vi "Master Setup Get Label and Pattern.vi"(2 "Use Master Setup":bool, 3 "Master Setup Patten Enum":i32(ring) items=["Channel Setup (0)", "PID Setup (1)", "Filter Setup (2)", "CAN Message Setup (3)", "CAN 1 Setup (4)", "CAN 2 Setup (5)", "Digital Inputs Setup (6)", "Digital Outputs Setup (7)", "Logging 1 Setup (8)", "Logging 2 Setup (9)", "Logging 3 Setup (10)", "Setpoint Setup (11)", "Test Series Setup (12)", "Graph Setup (13)", "System Configure (14)", "Header (15)", "Profile Manager (16)", "Post-Mortem Logging (17)", "High-Speed Data (18)", "Statistic Channel Setup (19)", "Ramp Channel Setup (20)", "ETAS INCA Channel Setup (21)", "ETC ECCS Transducer Setup (22)", "ETC ECCS Test Setup (23)", "AVL AK Smoke Meter Setup (24)", "Triggers Setup (25)", "Alarm Limits Setup (26)", "YKWT1 Measurement (27)", "YKWT1 Instrument (28)", "Auto File Settings (29)", "Playback File Setting (30)", "UUT Constants (31)", "UPS Setup (32)", "Differential Channel Setup (33)", "Integral Channel Setup (34)", "Signal Channel Setup (35)", "Calibration Setup (36)", "BNC Setup (37)", "ASAP3 Setup (38)", "Chassis Force Calculations (39)", "Chassis Teststand Losses (40)", "Chassis Vehicle Losses (41)", "Formula Channels (42)", "ASAP3 Map Coords Setup (43)", "Digital Controls Setup (44)", "Push Buttons Setup (45)", "Sliders Setup (46)", "~Reserved~ (47)", "Email Setup (48)", "Timer Setup (49)", "Unit Conversion Setup (50)", "Visible Channels (51)", "Main Display Setup (52)", "Message Display Setup (53)", "Input Display Setup (54)", "Unico Parameter Downloads (55)", "Flow Meter Setup (56)", "Channel Zero Offset (57)", "YKWT2 Measurement (58)", "YKWT2 Instrument (59)", "CAN 3 Setup (60)", "CAS Setup (61)", "Accumulation Channel Setup (62)", "Valvetrain Dynamics Setup (63)", "CCP Setup (64)", "System Log Setup (65)", "Throttle Controller (66)", "RE Shifter (67)", "Main Display (68)", "~Reserved~ (69)", "FlexRay (70)"]) -> (0 "Pattern Label":string, 1 "Pattern":string)   [LabVIEW 2017]
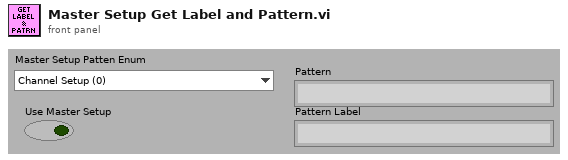
[diagram p1: front panel]
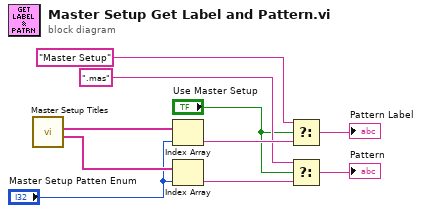
[diagram p0: block diagram]
diagram:
  n1 = call "Master Setup Titles.vi"() -> ("Setup Patterns"=w10:string[], "Setup Description"=w9:string[])  [unwired: 6 in, 4 out]
  n2 = Index Array(array=w9, index="Master Setup Patten Enum") -> (element=w8:string)
  n3 = Index Array(array=w10, index="Master Setup Patten Enum") -> (element=w7:string)
  n4 = Select(t="Master Setup", s="Use Master Setup", f=w8) -> (s? t:f=→"Pattern Label":string)
  n5 = Select(t=".mas", s="Use Master Setup", f=w7) -> (s? t:f=→"Pattern":string)
